vi "Setup_CHROMA_nestec.vi"() -> (1 "Frequency CHROMA display":dbl, 2 "Voltage CHROMA display":dbl)   [LabVIEW 2014]
panel:
  out "error out":errorcluster
  in  "Preset":u16(ring) items=["STOP", "230 V / 50 Hz", "120 V / 60 Hz", "100 V / 60 Hz"]
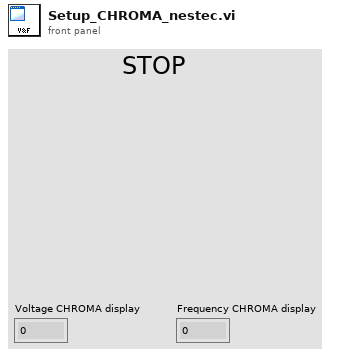
[diagram p1: front panel]
types:
  T1 = enum8{"Enabled", "Disabled", "Disabled and Grayed Out"}
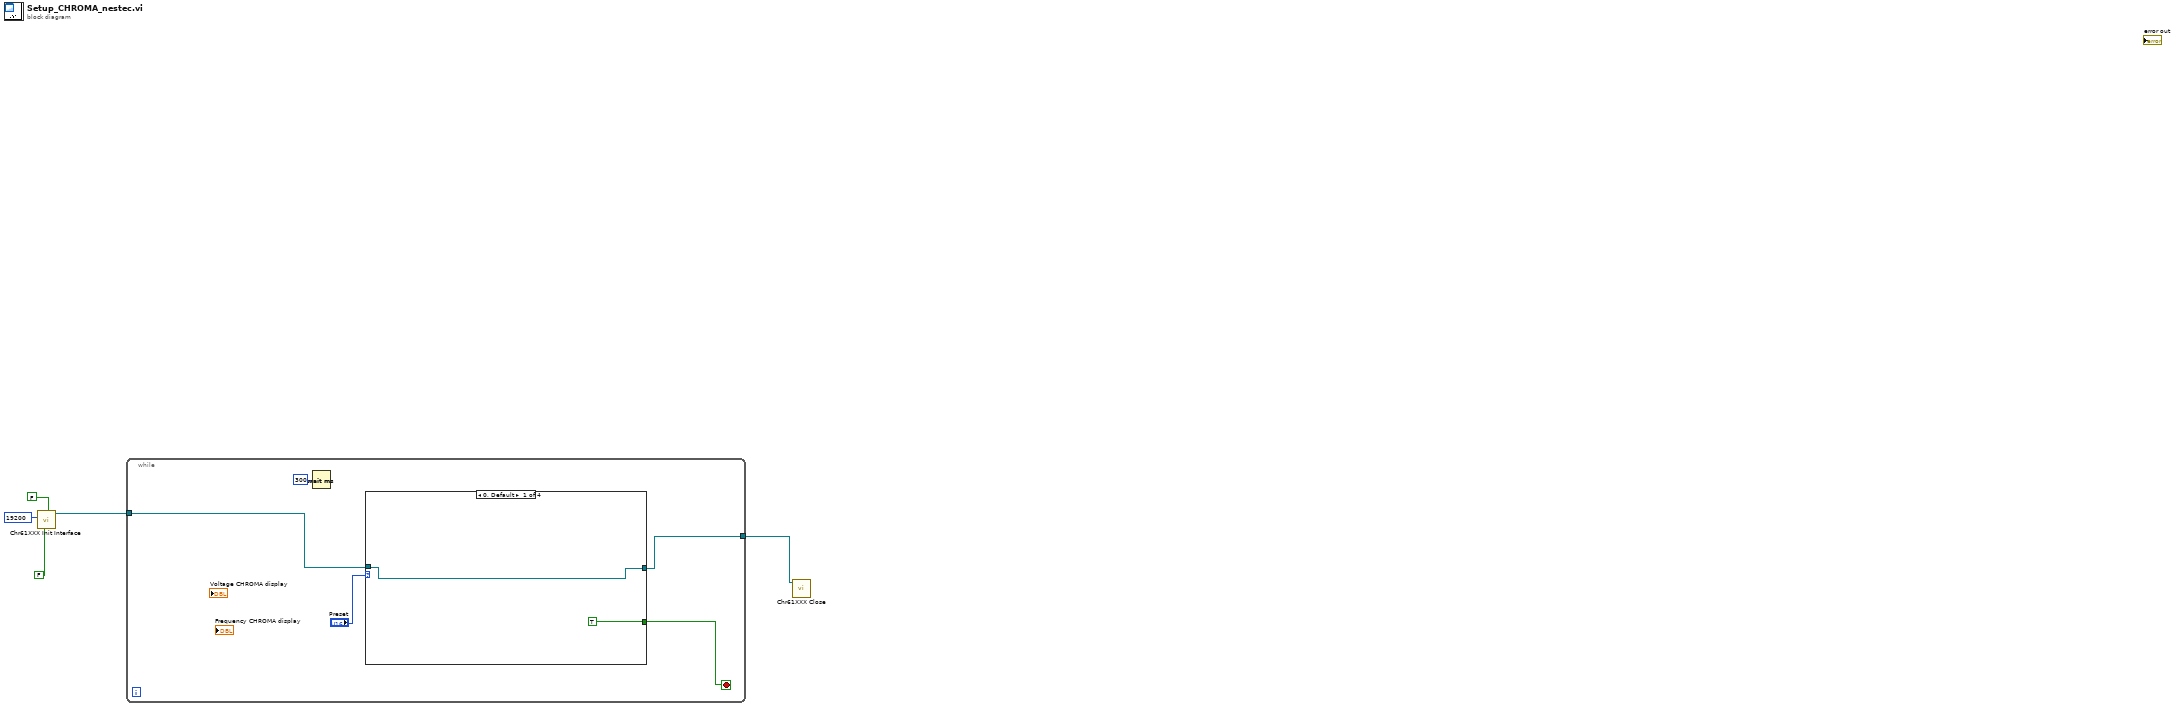
[diagram p0: block diagram]
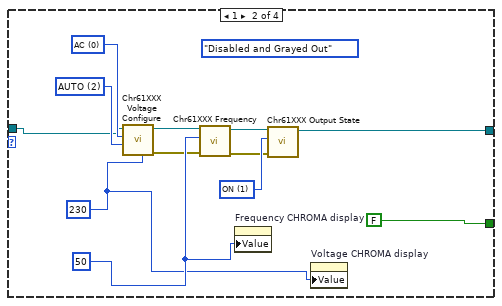
[diagram p2: hidden frame]
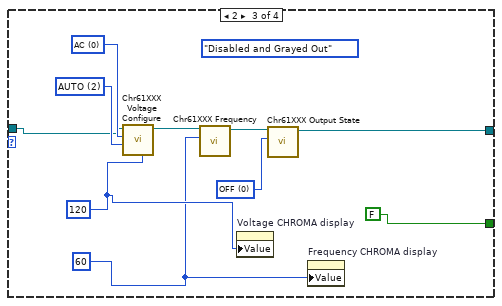
[diagram p3: hidden frame]
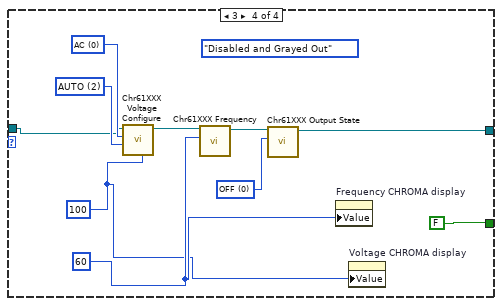
[diagram p4: hidden frame]
diagram:
  w3 = 19200 items=["9600"=9600, "19200"=19200, "38400"=38400, "57600"=57600, "115200"=115200] ("baud rate")
  n1 = call <instrlib>:"Chr61XXX Init Interface.vi"("id query"=FALSE, "reset device"=FALSE, "baud rate"=w3) -> ("instrument handle out"=w5:refnum<k15>)  [unwired: 6 in, 2 out]
  n2 = while {
    tunnel: w5 -> [w10]
    tunnel: [w9] -> w4
    stop <- w8 stop-if-true
    n3 = Wait (ms)(milliseconds to wait=u32 300) -> ()  [unwired: 1 out]
    n4 = case shown="0, Default" "Preset" {
      tunnel: w10 -> [w12 w18 w28 w39]
      tunnel: [w12 w19 w29 w38] -> w9
      tunnel: [TRUE FALSE FALSE FALSE] -> w8
      frame 0, Default {
      }
      frame 1 {
        w16 = 50
        w15 = 230
        (unwired) T1."Disabled and Grayed Out" ("Disabled")
        w24 = 2 items=["LOW", "HIGH", "AUTO"] ("voltage range")
        w23 = 0 items=["AC", "DC"] ("voltage type")
        w20 = u16 1 items=["OFF", "ON"] ("state")
        n5 = call <instrlib>:"Chr61XXX Voltage Configure.vi"("voltage"=w15, "voltage range"=w24, "voltage type"=w23, "instrument handle"=w18) -> ("error out"=w14:errorcluster, "instrument handle out"=w22:refnum<k15>)  [unwired: 6 in]
        n6 = call <instrlib>:"Chr61XXX Frequency.vi"("error in (no error)"=w14, "frequency"=w16, "instrument handle"=w22) -> ("error out"=w13:errorcluster, "instrument handle out"=w21:refnum<k15>)  [unwired: 7 in]
        n7 = property on="Frequency CHROMA display" class="DigNum (strict)"("Value"=w16) -> ()  [unwired: 2 in, 2 out]
        n8 = call <instrlib>:"Chr61XXX Output State.vi"("error in (no error)"=w13, "state"=w20, "instrument handle"=w21) -> ("instrument handle out"=w19:refnum<k15>)  [unwired: 7 in, 1 out]
        n9 = property on="Voltage CHROMA display" class="DigNum (strict)"("Value"=w15) -> ()  [unwired: 2 in, 2 out]
      }
      frame 2 {
        w25 = 60
        w26 = 120
        (unwired) T1."Disabled and Grayed Out" ("Disabled")
        w34 = 2 items=["LOW", "HIGH", "AUTO"] ("voltage range")
        w33 = 0 items=["AC", "DC"] ("voltage type")
        w30 = u16 0 items=["OFF", "ON"] ("state")
        n10 = call <instrlib>:"Chr61XXX Voltage Configure.vi"("voltage"=w26, "voltage range"=w34, "voltage type"=w33, "instrument handle"=w28) -> ("instrument handle out"=w32:refnum<k15>)  [unwired: 6 in, 1 out]
        n11 = call <instrlib>:"Chr61XXX Frequency.vi"("frequency"=w25, "instrument handle"=w32) -> ("instrument handle out"=w31:refnum<k15>)  [unwired: 8 in, 1 out]
        n12 = property on="Voltage CHROMA display" class="DigNum (strict)"("Value"=w26) -> ()  [unwired: 2 in, 2 out]
        n13 = call <instrlib>:"Chr61XXX Output State.vi"("state"=w30, "instrument handle"=w31) -> ("instrument handle out"=w29:refnum<k15>)  [unwired: 8 in, 1 out]
        n14 = property on="Frequency CHROMA display" class="DigNum (strict)"("Value"=w25) -> ()  [unwired: 2 in, 2 out]
      }
      frame 3 {
        w36 = 60
        w35 = 100
        (unwired) T1."Disabled and Grayed Out" ("Disabled")
        w44 = 2 items=["LOW", "HIGH", "AUTO"] ("voltage range")
        w43 = 0 items=["AC", "DC"] ("voltage type")
        w40 = u16 0 items=["OFF", "ON"] ("state")
        n15 = call <instrlib>:"Chr61XXX Voltage Configure.vi"("voltage"=w35, "voltage range"=w44, "voltage type"=w43, "instrument handle"=w39) -> ("instrument handle out"=w42:refnum<k15>)  [unwired: 6 in, 1 out]
        n16 = call <instrlib>:"Chr61XXX Frequency.vi"("frequency"=w36, "instrument handle"=w42) -> ("instrument handle out"=w41:refnum<k15>)  [unwired: 8 in, 1 out]
        n17 = call <instrlib>:"Chr61XXX Output State.vi"("state"=w40, "instrument handle"=w41) -> ("instrument handle out"=w38:refnum<k15>)  [unwired: 8 in, 1 out]
        n18 = property on="Frequency CHROMA display" class="DigNum (strict)"("Value"=w36) -> ()  [unwired: 2 in, 2 out]
        n19 = property on="Voltage CHROMA display" class="DigNum (strict)"("Value"=w35) -> ()  [unwired: 2 in, 2 out]
      }
    }
  }
  n20 = call <instrlib>:"Chr61XXX Close.vi"("instrument handle"=w4) -> ()  [unwired: 10 in, 1 out]
